vi "example-rx-c-api.vi"() -> ()   [LabVIEW 2024]
uses:
  uhd (generated from wizard into user.lib - manually fixed for rx example)/uhd.lvlib
panel:
  in  "drop initial samples":i32=20000
  in  "ant":string="RX2"
  out "ant_out out":string="RX2"
  out "Waveform Graph":sgl[][](graph)
  out "items_recvd (sum)":u64=1020000
  out "error out":errorcluster
  out "items_recvd":u64=2040
  in  "num_samps":u64=1000000
  out "freq_out out":dbl=1000000000.0 format="%#_6p"
  in  "target_freq":dbl=1000000000.0 format="%#_6p"
  out "gain_out out":dbl
  in  "gain":dbl
  out "rate_out out":dbl=1000000.0 format="%#_6p"
  in  "chan":u64
  in  "rate":dbl=1000000.0 format="%#_6p"
  in  "args":string="type=b200"
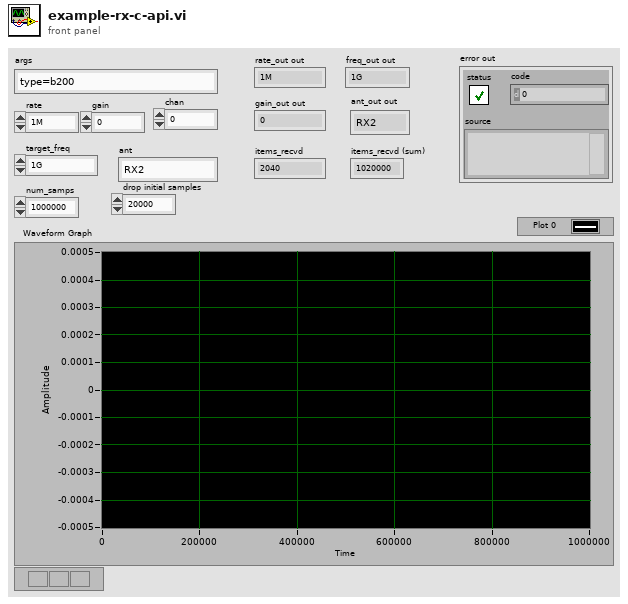
[diagram p1: front panel]
types:
  T1 = cluster{"stream_mode":u32, "@dummy control@":i8, "@dummy control@":i8, "@dummy control@":i8, "@dummy control@":i8, "num_samps":u64, "stream_now":i32, "@dummy control@":i8, "@dummy control@":i8, "@dummy control@":i8, "@dummy control@":i8, "time_spec_full_secs":i64, "time_spec_frac_secs":dbl}
  T2 = cluster{"cpu_format":string, "otw_format":string, "args":string, "channel_list":u64[], "n_channels":i32}
  T3 = cluster{"target_freq":dbl, "rf_freq_policy":u32, "@dummy control@":i8, "@dummy control@":i8, "@dummy control@":i8, "@dummy control@":i8, "rf_freq":dbl, "dsp_freq_policy":u32, "@dummy control@":i8, "@dummy control@":i8, "@dummy control@":i8, "@dummy control@":i8, "dsp_freq":dbl, "args":u64}
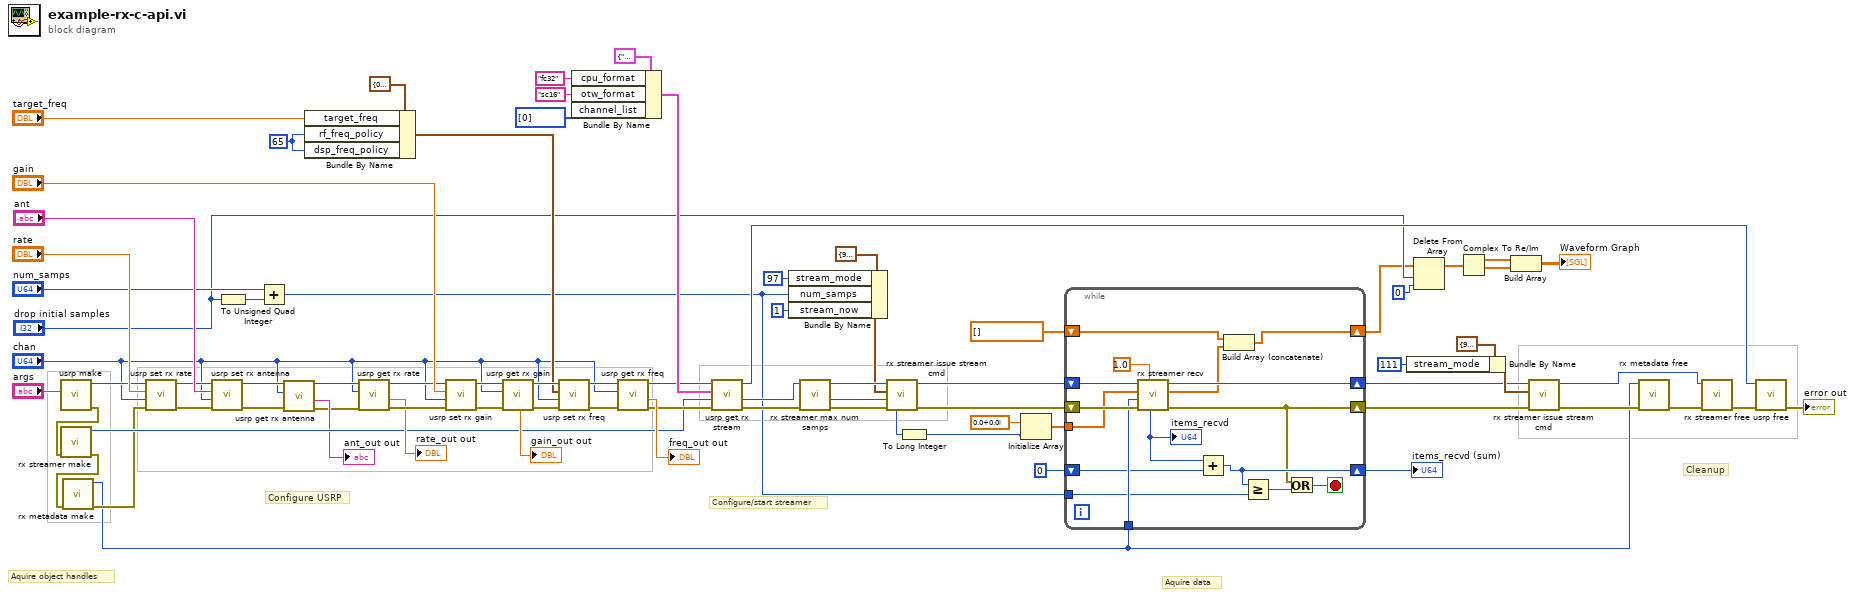
[diagram p0: block diagram]
diagram:
  w62 = u32 65 ("rf_freq_policy")
  # "Cleanup"
  # "Aquire data"
  # "Configure/start streamer"
  # "Configure USRP"
  # "Aquire object handles"
  n1 = call "usrp make.vi"("args"="args") -> ("error out"=w76:errorcluster, "h"=w37:u64)  [unwired: 8 in, 1 out]
  n2 = call "rx streamer make.vi"("error in (no error)"=w76) -> ("error out"=w75:errorcluster, "h 3"=w34:u64)  [unwired: 8 in, 1 out]
  n3 = call "rx metadata make.vi"("error in (no error)"=w75) -> ("error out"=w10:errorcluster, "handle out"=w1:u64)  [unwired: 8 in, 1 out]
  n4 = call "usrp set rx rate.vi"("error in (no error)"=w10, "chan"="chan", "rate"="rate", "h"=w37) -> ("error out"=w23:errorcluster, "h 2"=w27:u64)  [unwired: 5 in, 1 out]
  n5 = call "usrp set rx antenna.vi"("error in (no error)"=w23, "chan"="chan", "ant"="ant", "h"=w27) -> ("error out"=w25:errorcluster, "h 2"=w26:u64)  [unwired: 5 in, 1 out]
  n6 = To Unsigned Quad Integer(1:"drop initial samples") -> (0:w15:u64)
  n7 = Add(x="num_samps", y=w15) -> (x+y=w16:u64)
  n8 = call "usrp get rx antenna.vi"("error in (no error)"=w25, "chan"="chan", "h"=w26) -> ("error out"=w22:errorcluster, "ant_out out"=→"ant_out out":string)  [unwired: 5 in, 2 out]
  n9 = Bundle By Name(cluster=T3 {"target_freq"=0.0, "rf_freq_policy"=65, "@dummy control@"=0, "@dummy control@"=0, "@dummy control@"=0, "@dummy control@"=0, "rf_freq"=0.0, "dsp_freq_policy"=65, "@dummy control@"=0, "@dummy control@"=0, "@dummy control@"=0, "@dummy control@"=0, "dsp_freq"=0.0, "args"=0} ("tune_request"), "target_freq"="target_freq", "rf_freq_policy"=w62, "dsp_freq_policy"=w62) -> (w61:T3)
  n10 = call "usrp get rx rate.vi"("error in (no error)"=w22, "chan"="chan", "h"=w27) -> ("error out"=w73:errorcluster, "rate_out out"=→"rate_out out":dbl, "h 2"=w68:u64)  [unwired: 5 in, 1 out]
  n11 = call "usrp set rx gain.vi"("error in (no error)"=w73, "chan"="chan", "gain"="gain", "h"=w68) -> ("error out"=w70:errorcluster, "h 2"=w69:u64)  [unwired: 5 in, 1 out]
  n12 = call "usrp get rx gain.vi"("error in (no error)"=w70, "chan"="chan", "h"=w69) -> ("error out"=w65:errorcluster, "h 2"=w66:u64, "gain_out out"=→"gain_out out":dbl)  [unwired: 5 in, 1 out]
  n13 = call "usrp set rx freq.vi"("error in (no error)"=w65, "chan"="chan", "tune_request"=w61, "h"=w66) -> ("error out"=w59:errorcluster, "h 3"=w60:u64)  [unwired: 2 in, 4 out]
  n14 = Bundle By Name(cluster=T2 {"cpu_format"="", "otw_format"="", "args"="", "channel_list"=[], "n_channels"=0} ("stream_args"), "cpu_format"="fc32", "otw_format"="sc16", "channel_list"=u64[] [0]) -> (w52:T2)
  n15 = call "usrp get rx freq.vi"("error in (no error)"=w59, "chan"="chan", "h"=w60) -> ("error out"=w57:errorcluster, "freq_out out"=→"freq_out out":dbl, "h 2"=w35:u64)  [unwired: 5 in, 1 out]
  n16 = call "usrp get rx stream.vi"("error in (no error)"=w57, "h 3"=w34, "stream_args"=w52, "h"=w35) -> ("error out"=w51:errorcluster, "h 4"=w36:u64, "h 2"=w38:u64)  [unwired: 3 in, 2 out]
  n17 = Bundle By Name(cluster=T1 {"stream_mode"=97, "@dummy control@"=0, "@dummy control@"=0, "@dummy control@"=0, "@dummy control@"=0, "num_samps"=0, "stream_now"=0, "@dummy control@"=0, "@dummy control@"=0, "@dummy control@"=0, "@dummy control@"=0, "time_spec_full_secs"=0, "time_spec_frac_secs"=0.0} ("stream_cmd"), "stream_mode"=u32 97, "num_samps"=w16, "stream_now"=1) -> (w46:T1)
  n18 = call "rx streamer max num samps.vi"("error in (no error)"=w51, "h"=w36) -> ("error out"=w49:errorcluster, "max_num_samps_out out"=w33:u64, "h 2"=w50:u64)  [unwired: 6 in, 1 out]
  n19 = call "rx streamer issue stream cmd.vi"("error in (no error)"=w49, "stream_cmd"=w46, "h"=w50) -> ("error out"=w9:errorcluster, "h 2"=w45:u64)  [unwired: 6 in, 1 out]
  n20 = To Long Integer(number=w33) -> (32bit integer=w20:i32)
  n21 = Initialize Array(csg 0.0+0.0i ("single precision complex"), w20) -> (w18:csg[])
  n22 = while {
    tunnel: w1 -> [w92]
    tunnel: w18 -> [w91]
    shift-right: [w80] -> w8
    shift-left: w9 -> [w93]
    shift-right: [w88] -> w41
    shift-left: w45 -> [w90]
    shift-right: [w85] -> w29
    shift-left: u64 0 ("items_recvd out") -> [w86]
    tunnel: w16 -> [w84]
    shift-right: [w81] -> w13
    shift-left: csg[] [] ("buffs out") -> [w83]
    stop <- w78 stop-if-true
    n23 = call "rx streamer recv.vi"("timeout"=1.0, "error in (no error)"=w93, "md"=w92, "buffs"=w91, "h"=w90) -> ("error out"=w80:errorcluster, "buffs out"=w82:csg[], "h 2"=w88:u64, "items_recvd out"=w87:u64)  [unwired: 1 in, 2 out]
    "items_recvd" <- w87
    n24 = Add(x=w87, y=w86) -> (x+y=w85:u64)
    n25 = Build Array (concatenate)(w83, w82) -> (w81:csg[])
    n26 = Greater Or Equal?(x=w85, y=w84) -> (x >= y?=w79:bool)
    n27 = Or(x=w80, y=w79) -> (x .or. y?=w78:bool)
  }
  "items_recvd (sum)" <- w29
  n28 = Bundle By Name(cluster=T1 {"stream_mode"=97, "@dummy control@"=0, "@dummy control@"=0, "@dummy control@"=0, "@dummy control@"=0, "num_samps"=0, "stream_now"=0, "@dummy control@"=0, "@dummy control@"=0, "@dummy control@"=0, "@dummy control@"=0, "time_spec_full_secs"=0, "time_spec_frac_secs"=0.0} ("stream_cmd"), "stream_mode"=u32 111) -> (w42:T1)
  n29 = Delete From Array(array=w13, length="drop initial samples", index=0) -> (array with subset deleted=w12:csg[])  [unwired: 1 out]
  n30 = Complex To Re/Im(x + iy=w12) -> (x=w6:sgl[], y=w7:sgl[])
  n31 = Build Array(w6, w7) -> (→"Waveform Graph":sgl[][])
  n32 = call "rx streamer issue stream cmd.vi"("error in (no error)"=w8, "stream_cmd"=w42, "h"=w41) -> ("error out"=w40:errorcluster, "h 2"=w39:u64)  [unwired: 6 in, 1 out]
  n33 = call "rx metadata free.vi"("error in (no error)"=w40, "handle"=w1) -> ("error out"=w4:errorcluster)  [unwired: 7 in, 2 out]
  n34 = call "rx streamer free.vi"("error in (no error)"=w4, "h"=w39) -> ("error out"=w3:errorcluster)  [unwired: 7 in, 2 out]
  n35 = call "usrp free.vi"("error in (no error)"=w3, "h"=w38) -> ("error out"=→"error out":errorcluster)  [unwired: 7 in, 2 out]
